vi "test_RLSE.vi"() -> ()   [LabVIEW 2021]
uses:
  <vilib>/Analysis/Matrix/Datatypes/RealMatrix.ctl
  <vilib>/Analysis/Matrix/NI_Matrix.lvlib
  <vilib>/Analysis/NI_AALBase.lvlib
panel:
  out "Waveform Chart":dbl[](graph)
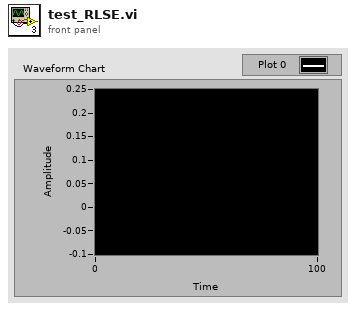
[diagram p1: front panel]
types:
  T1 = typedef "NI_Matrix.lvlib/RealMatrix.ctl" = dbl[][]
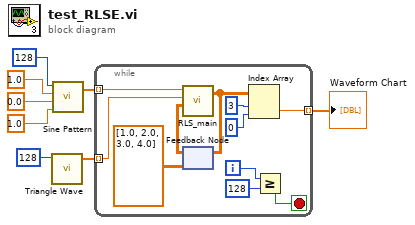
[diagram p0: block diagram]
diagram:
  n1 = call <vilib>:"Triangle Wave.vi"("samples"=128) -> ("triangle wave"=w3:dbl[])  [unwired: 4 in, 2 out]
  n2 = call <vilib>:"Sine Pattern.vi"("cycles"=1.0, "phase(degrees)"=0.0, "amplitude"=1.0, "samples"=128) -> ("Sinusoidal Pattern"=w8:dbl[])  [unwired: 1 out]
  n3 = while {
    tunnel: w8 -> [w17] mode=indexing
    tunnel: w3 -> [w16] mode=indexing
    tunnel: [w12] -> w2 mode=indexing
    i -> [w11]
    stop <- w9 stop-if-true
    n4 = feedback #1(T1 [[1.0], [2.0], [3.0], [4.0]] ("\\theta (t)")) -> (w18:T1)
    n5 = call "RLS_main.vi"("\\theta (t-1)"=w18, "u(t)"=w16, "x(t)"=w17) -> ("\\theta (t)"=w15:T1)  [unwired: 1 in, 1 out]
    n6 = feedback-in #1(w15) -> ()
    n7 = Index Array(array=w15, index (row)=3, index (col)=0) -> (element=w12:dbl)
    n8 = Greater Or Equal?(x=w11, y=128) -> (x >= y?=w9:bool)
  }
  "Waveform Chart" <- w2
